vi "liste valves expediées en txt.vi"(1 "Tab valves":string[][](array[string])=[["12-216C-04520 EQIFIL 104mA 36ohm", "112105740008030110", "18.04.2008 15:35", "MQI", "12345/06-03.03.03", "2", "30"], ["12-216C-04520 EQIFIL 104mA 36ohm", "112105740008030109", "18.04.2008 15:35", "MQI", "12345/06-03.03.03", "2", "30"], ["12-216C-04520 EQIFIL 104mA 36ohm", "112105740008030108", "18.04.2008 15:35", "MQI", "12345/06-03.03.03", "2", "30"], ["12-216C-04520 EQIFIL 104mA 36ohm", "112105740008030107", "18.04.2008 15:35", "MQI", "12345/06-03.03.03", "1", "30"], ["12-216C-04520 EQIFIL 104mA 36ohm", "112105740008030106", "18.04.2008 15:35", "MQI", "12345/06-03.03.03", "1", "30"], ["12-216C-04520 EQIFIL 104mA 36ohm", "112105740008030105", "18.04.2008 15:35", "MQI", "12345/06-03.03.03", "1", "30"], ["12-216C-04520 EQIFIL 104mA 36ohm", "112105740008030104", "18.04.2008 15:35", "MQI", "12345/06-03.03.03", "1", "30"], ["12-216C-04520 EQIFIL 104mA 36ohm", "112105740008030103", "18.04.2008 15:35", "MQI", "12345/06-03.03.03", "1", "30"], ["12-216C-04520 EQIFIL 104mA 36ohm", "112105740008030102", "18.04.2008 15:35", "MQI", "12345/06-03.03.03", "1", "30"], ["12-216C-04520 EQIFIL 104mA 36ohm", "112105740008030101", "18.04.2008 15:35", "MQI", "12345/06-03.03.03", "1", "30"]]) -> (0 "liste valves":string="Carton : 1/2\r112105740008030107\r112105740008030106\r112105740008030105\r112105740008030104\r112105740008030103\r112105740008030102\r112105740008030101\r\rCarton : 2/2\r112105740008030110\r112105740008030109\r112105740008030108\r\r")   [LabVIEW 2020]
doc: "Mise en forme txt de la liste des valves emballées par carton pour aller dans la pièce jointe du mail expédition."
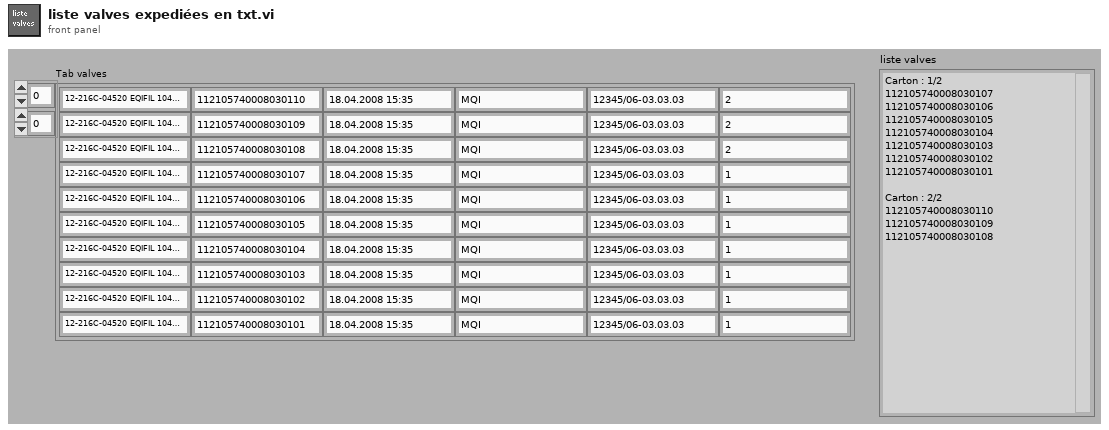
[diagram p1: front panel]
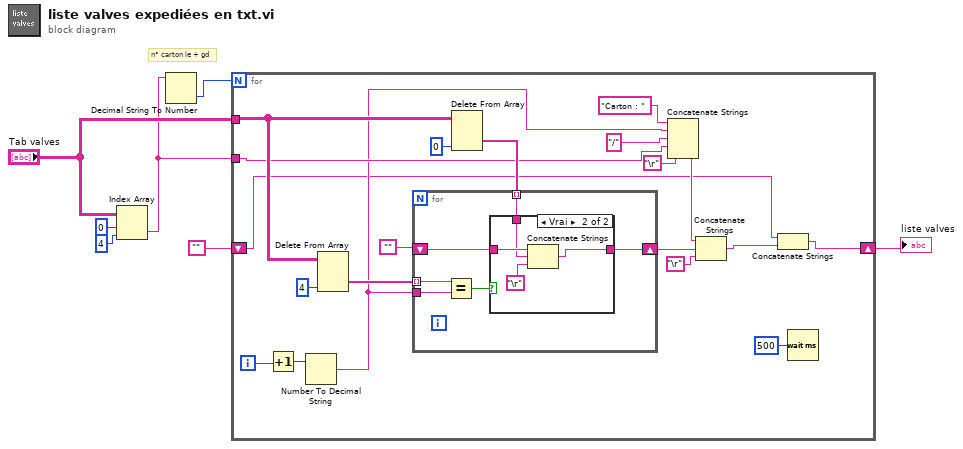
[diagram p0: block diagram]
diagram:
  # "n° carton le + gd"
  n1 = Index Array(array="Tab valves", index (row)=0 ("indice désactivé (ligne)"), index (col)=4 ("indice désactivé (col)")) -> (element=w4:string)
  n2 = Decimal String To Number(string=w4) -> (number=w1:i32)  [unwired: 2 in, 1 out]
  n3 = for {
    N: w1 -> [_]
    tunnel: "Tab valves" -> [w22]
    tunnel: w4 -> [w16]
    shift-right: [w10] -> w2
    shift-left: "" -> [w9]
    i -> [w21]
    n4 = Increment(x=w21) -> (x+1=w27:i32)
    n5 = Number To Decimal String(number=w27) -> (decimal integer string=w15:string)  [unwired: 1 in]
    n6 = Delete From Array(array=w22, index (col)=4 ("indice désactivé (col)")) -> (deleted portion=w24:string[])  [unwired: 2 in, 1 out]
    n7 = Delete From Array(array=w22, index (col)=0 ("indice désactivé (col)")) -> (deleted portion=w26:string[])  [unwired: 2 in, 1 out]
    n8 = for {
      tunnel: w24 -> [w32] mode=indexing
      tunnel: w15 -> [w33]
      shift-right: [w29] -> w14
      shift-left: "" -> [w28]
      tunnel: w26 -> [w30] mode=indexing
      n9 = Equal?(x=w32, y=w33) -> (x = y?=w31:bool)
      n10 = case shown="Vrai" w31 {
        tunnel: w30 -> [_ w37]
        tunnel: [w34 w35] -> w29
        tunnel: w28 -> [w34 w38]
        frame False {
        }
        frame True {
          n11 = Concatenate Strings(w38, w37, "\r") -> (w35:string)
        }
      }
    }
    n12 = Concatenate Strings("Carton : " ("expression régulière"), w15, "/" ("chaîne"), w16, "\r") -> (w12:string)
    n13 = Concatenate Strings(w12, w14, "\r") -> (w11:string)
    n14 = Concatenate Strings(w9, w11) -> (w10:string)
    n15 = Wait (ms)(milliseconds to wait=u32 500 ("attente (ms)")) -> ()  [unwired: 1 out]
  }
  "liste valves" <- w2
